vi "Clear Symbol Map.vi"(8 "error in (no error)":errorcluster, 11 "TwinCAT ADS in":refnum<class "TwinCAT ADS.lvclass">) -> (0 "error out":errorcluster, 3 "TwinCAT ADS out":refnum<class "TwinCAT ADS.lvclass">)   [LabVIEW 2018, in "TwinCAT ADS.lvclass"]
uses:
  TwinCAT ADS.lvclass
  TwinCAT ADS.lvclass/TwinCAT ADS.ctl
  TwinCAT.Ads
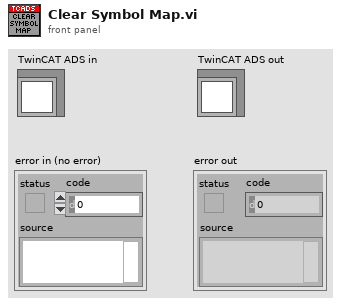
[diagram p1: front panel]
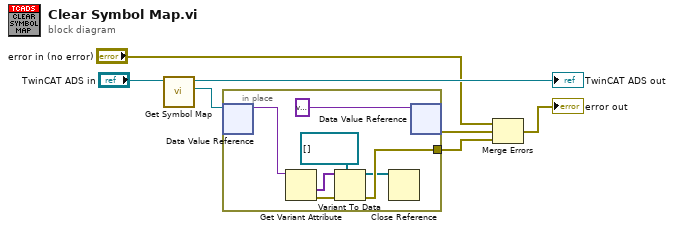
[diagram p0: block diagram]
diagram:
  n1 = call "Get Symbol Map.vi"("TwinCAT ADS in"="TwinCAT ADS in") -> ("Symbol Map"=w6:refnum<data-value>, "TwinCAT ADS out"=→"TwinCAT ADS out":refnum<class "TwinCAT ADS.lvclass">)  [unwired: 8 in, 1 out]
  n2 = in-place {
    in-place-border: [w9] -> w4
    n3 = in-place-dvr #1(w6) -> (w13:variant)  [unwired: 1 out]
    n4 = Get Variant Attribute(Variant=w13) -> (values=w11:variant[], error out=w12:errorcluster)  [unwired: 3 in, 2 out]
    n5 = Variant To Data(error in=w12, type=refnum<k24>[] [], Variant=w11) -> (data=w8:refnum<k24>[], error out=w9:errorcluster)
    n6 = Close Reference(reference=w8) -> ()  [unwired: 1 in, 1 out]
    n7 = in-place-dvr #1(variant ("data value")) -> (w3:errorcluster)  [unwired: 1 out]
  }
  n8 = Merge Errors("error in (no error)", w3, w4) -> (→"error out":errorcluster)
